vi "MeasureOAM.vi"() -> ()   [LabVIEW 2015]
uses:
  <vilib>/Utility/file.llb/Write Delimited Spreadsheet (DBL).vi
panel:
  out "SLM  B":picture
  out "SLM A":picture
  out "Calibration Curve":dbl[](array[numeric])=[1.04866638e-09, 2.36400149e-10, 3.28397032e-10, 3.4456285e-11, 1.42615789e-11, 6.36260558e-11, 1.65061454e-11, 1.20186092e-11, 3.22117194e-11, 4.34313557e-11, 1.69085523e-10, -3.68856204e-12, 5.28650778e-12, -1.44559289e-12, 7.52947704e-12, 3.04194213e-12, 9.77404269e-12, 3.04194213e-12, 7.52947704e-12, 7.98972867e-13, 3.04194213e-12]
  out "Measured Power":dbl=1.53557755e-09
  out "Generated OAM Progress":u8(slide)=100 scale=0.0..100.0
  out "Current Measured OAM":i32=10
  in  "Measured OAM":i32[](array[numeric])=[-10, -9, -8, -7, -6, -5, -4, -3, -2, -1, 0, 1, 2, 3, 4, 5, 6, 7, 8, 9, 10]
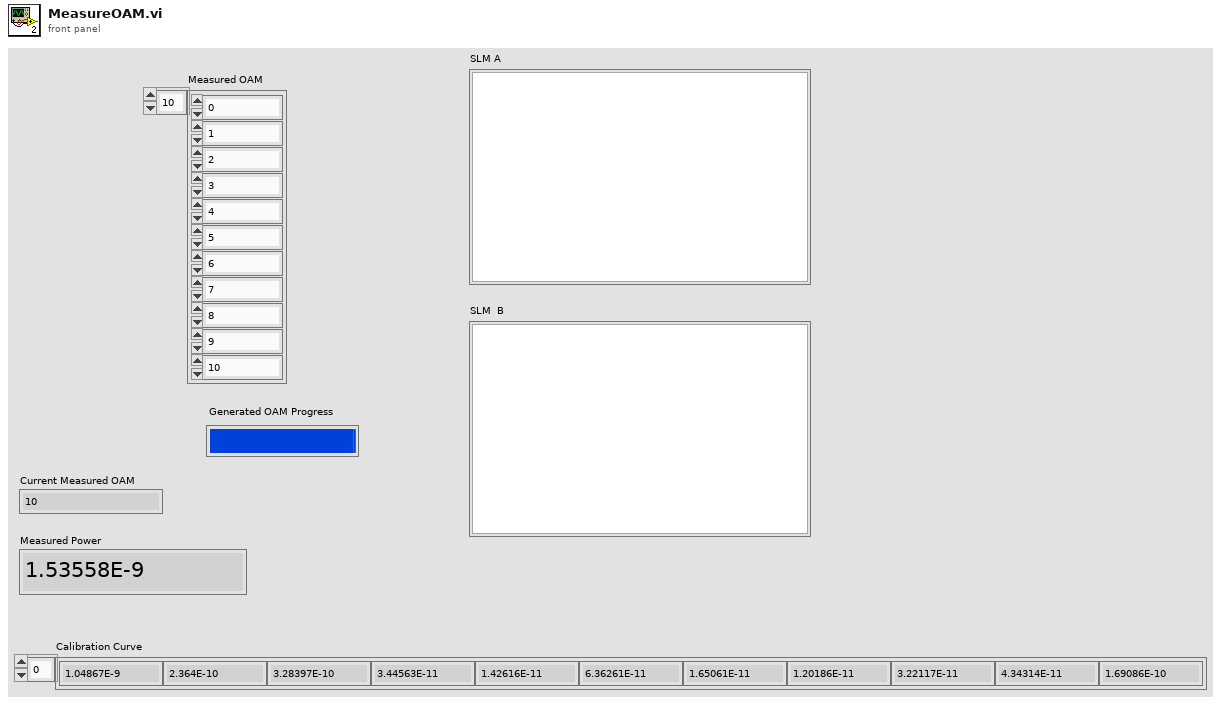
[diagram p1: front panel]
types:
  T1 = cluster{"type":enum16{"Azimuth Mode", "LG mode", "HG mode"}, i32, i32, dbl, dbl}
  T2 = cluster{"type":enum16{"Azimuth Mode", "LG mode", "HG mode"}, i32, i32, dbl, dbl}[]
  T3 = cluster{"type":enum16{"Azimuth Mode", "LG mode", "HG mode"}, "Numeric":i32, i32, dbl, dbl}
  T4 = cluster{"type":enum16{"Azimuth Mode", "LG mode", "HG mode"}, "Numeric":i32, i32, dbl, dbl}[]
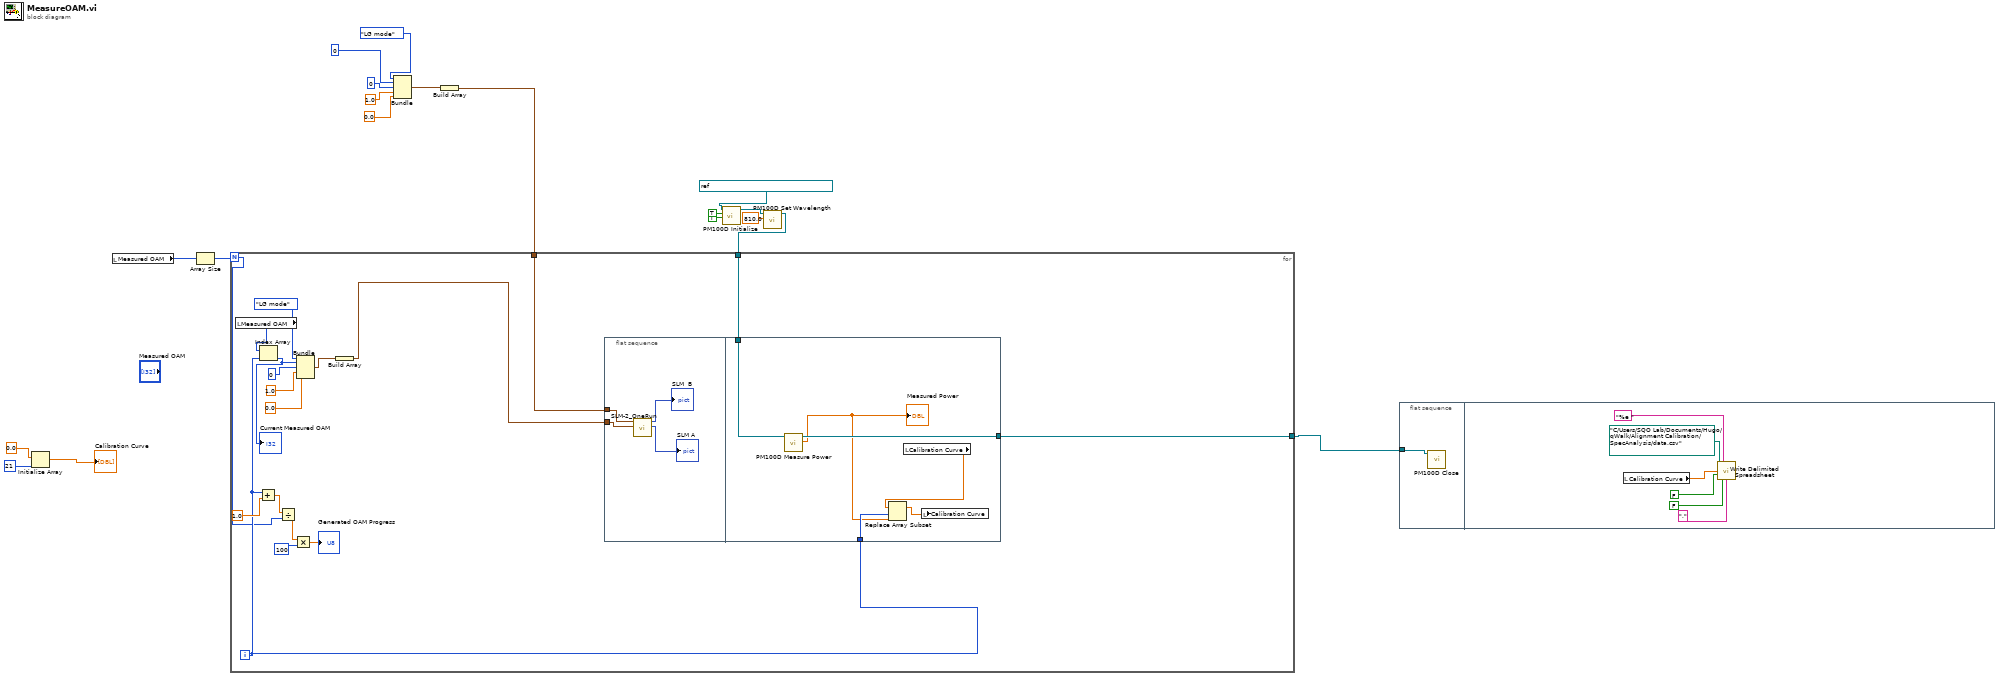
[diagram p0: block diagram]
diagram:
  n1 = Initialize Array(0.0 ("element"), 21 ("dimension size")) -> (→"Calibration Curve":dbl[])
  n2 = local read "Measured OAM"() -> (w19:i32[])
  n3 = Array Size(array=w19) -> (size(s)=w18:i32)
  n4 = Bundle("type"=enum16{"Azimuth Mode", "LG mode", "HG mode"}."LG mode", 0, 0, 1.0, 0.0) -> (w2:T1)  [unwired: 1 in]
  n5 = Build Array(w2) -> (w1:T2)
  n6 = call <instrlib>:"PM100D Initialize.vi"("Reset Device (Reset Device)"=TRUE, "ID Query (Do Query)"=TRUE, "resource name"=refnum<visa-resource-name> "USB0::0x1313::0x8078::P0014115::INSTR") -> ("instrument handle out"=w16:refnum<visa-resource-name>)  [unwired: 7 in, 1 out]
  n7 = call <instrlib>:"PM100D Set Wavelength.vi"("Wavelength (0.0)"=810.0, "instrument handle"=w16) -> ("instrument handle out"=w12:refnum<visa-resource-name>)  [unwired: 8 in, 1 out]
  n8 = for {
    N: w18 -> [w22]
    tunnel: w12 -> [w27]
    tunnel: [w26] -> w8
    tunnel: w1 -> [w20]
    i -> [w24]
    n9 = local read "Measured OAM"() -> (w37:i32[])
    n10 = Add(x=w24, y=1.0) -> (x+y=w23:dbl)
    n11 = Index Array(array=w37, index=w24) -> (element=w32:i32)
    "Current Measured OAM" <- w32
    n12 = Divide(x=w23, y=w22) -> (x/y=w21:dbl)
    n13 = Multiply(x=w21, y=100) -> (x*y=→"Generated OAM Progress":dbl)
    n14 = Bundle("type"=enum16{"Azimuth Mode", "LG mode", "HG mode"}."LG mode", "Numeric"=w32, 0, 1.0, 0.0) -> (w29:T3)  [unwired: 1 in]
    n15 = Build Array(w29) -> (w28:T4)
    n16 = flat-sequence {
      tunnel: w28 -> [w41]
      tunnel: w20 -> [w38]
      tunnel: w24 -> [w45]
      tunnel: w27 -> [w44]
      tunnel: [w43] -> w26
      frame #0 {
        n17 = call "SLM-2_OneRun.vi"("Modes B - SLM 2"=w41, "Modes - UV"=w38) -> ("SLM"=→"SLM A":picture, "SLM  B"=→"SLM  B":picture)  [unwired: 8 in]
      }
      frame #1 {
        n18 = call <instrlib>:"PM100D Measure Power.vi"("instrument handle"=w44) -> ("Power"=w42:dbl, "instrument handle out"=w43:refnum<visa-resource-name>)  [unwired: 8 in, 1 out]
        "Measured Power" <- w42
        n19 = local read "Calibration Curve"() -> (w47:dbl[])
        n20 = Replace Array Subset(array=w47, new element=w42, index=w45) -> (w46:dbl[])
        n21 = local write "Calibration Curve"(w46) -> ()
      }
    }
  }
  n22 = flat-sequence {
    tunnel: w8 -> [w48]
    frame #0 {
      n23 = call <instrlib>:"PM100D Close.vi"("instrument handle"=w48) -> ()  [unwired: 10 in, 1 out]
    }
    frame #1 {
      n24 = local read "Calibration Curve"() -> (w49:dbl[])
      n25 = call-poly <vilib>:"Write Delimited Spreadsheet.vi"("file path (dialog if empty)"=path "C:/Users/SQO Lab/Documents/Hugo/qWalk/Alignment Calibration/SpecAnalysis/data.csv", "format (%.3f)"="%e ", "1D data"=w49, "append to file? (F)"=FALSE, "transpose? (F)"=FALSE, "delimiter (\\t)"=",") -> ()  [unwired: 8 in, 2 out]
    }
  }
